vi "Get Tag Content.vi"(8 "error in (no error)":errorcluster, 9 "tag index":i32, 11 "xml in":T1) -> (0 "error out":errorcluster, 1 "found?":bool, 2 "element content":string, 3 "xml out":T1)   [LabVIEW 2011]
uses:
  XML Structure - Cluster.ctl
  XML Tag Type - Enum.ctl
panel:
  # "This VI must be set to Subroutine Priority"
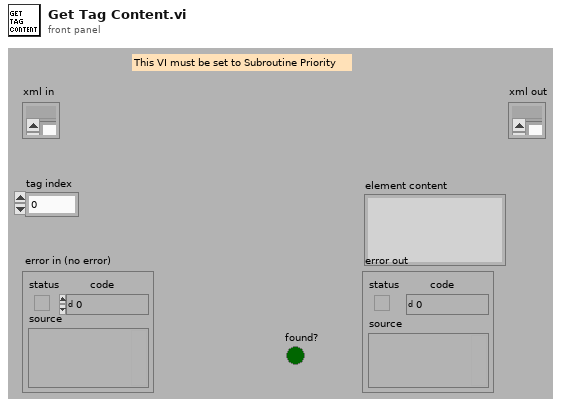
[diagram p1: front panel]
types:
  T1 = typedef "XML Structure - Cluster.ctl" = cluster{"tags":string[], "tag names":string[], "tag type":T2[], "offset":i32[], "close tag index":i32[], "xml":string, "Children":cluster{"children":i32[]}[], "parent index":i32[]}
  T2 = typedef "XML Tag Type - Enum.ctl" = enum16{"start tag", "empty tag", "end tag"}
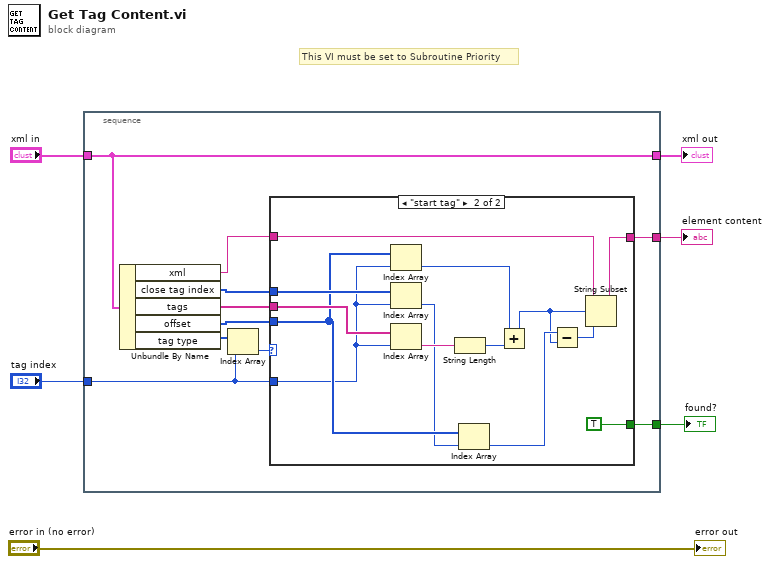
[diagram p0: block diagram]
diagram:
  # "This VI must be set to Subroutine Priority"
  n1 = stacked-sequence {
    tunnel: "xml in" -> [w11]
    tunnel: [w13] -> w4
    tunnel: "tag index" -> [w9]
    tunnel: [w11] -> w6
    tunnel: [w7] -> w1
    frame #0 {
      n2 = Unbundle By Name(w11) -> ("xml"=w12:string, "close tag index"=w16:i32[], "tags"=w15:string[], "offset"=w14:i32[], "tag type"=w10:T2[])
      n3 = Index Array(array=w10, index=w9) -> (element=w8:T2)
      n4 = case shown="\"start tag\"" w8 {
        tunnel: w16 -> [_ w30]
        tunnel: w15 -> [_ w29]
        tunnel: w14 -> [_ w27]
        tunnel: [_ w26] -> w13
        tunnel: w12 -> [_ w19]
        tunnel: w9 -> [_ w18]
        tunnel: [_ TRUE] -> w7
        frame Default {
        }
        frame "start tag" {
          n5 = Index Array(array=w27, index=w18) -> (element=w21:i32)
          n6 = Index Array(array=w30, index=w18) -> (element=w25:i32)
          n7 = Index Array(array=w29, index=w18) -> (element=w28:string)
          n8 = String Length(string=w28) -> (length=w22:i32)
          n9 = Index Array(array=w27, index=w25) -> (element=w23:i32)
          n10 = Add(x=w21, y=w22) -> (x+y=w20:i32)
          n11 = Subtract(x=w23, y=w20) -> (x-y=w24:i32)
          n12 = String Subset(string=w19, offset (0)=w20, length (rest)=w24) -> (substring=w26:string)
        }
      }
    }
  }
  "xml out" <- w6
  "element content" <- w4
  "found?" <- w1
  "error out" <- "error in (no error)"
